vi "Log Internal.vi"(9 "data (null)":variant, 10 "message":string, 11 "logger in":refnum<class "Logger.lvclass">) -> (3 "logger out":refnum<class "Logger.lvclass">)   [LabVIEW 2018, in "Logging.lvlib" / "Logger.lvclass"]
uses:
  Logger.lvclass
panel:
  # "Connector Pane"
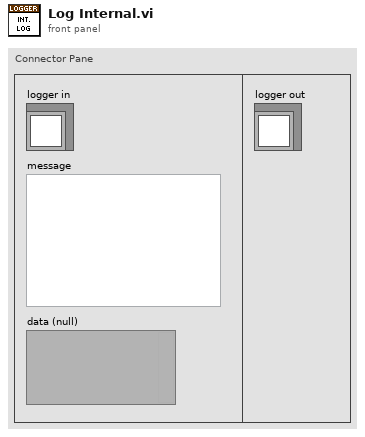
[diagram p1: front panel]
types:
  T1 = typedef "Logging.lvlib/Log Record.ctl" = cluster{"level":T2, "timestamp":timestamp, "call chain":string[], "message":string, "data":variant}
  T2 = typedef "Logging.lvlib/Internal Log Levels.ctl" = enum16{"Trace", "Debug", "Info", "Warning", "Error", "Critical", "Internal"}
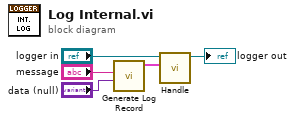
[diagram p0: block diagram]
diagram:
  n1 = call "Generate Log Record.vi"("data (null)"="data (null)", "message (\"\")"="message") -> ("log record"=w2:T1)  [unwired: 9 in]
  n2 = call "Handle.vi"("log record"=w2, "logger in"="logger in") -> ("logger out"=→"logger out":refnum<class "Logger.lvclass">)  [unwired: 9 in]
